vi "AWG Commit.vi"(8 "error in":errorcluster, 11 "Semiconductor Module Context In":T1) -> (0 "error out":errorcluster, 2 "Instruments Handle Out":refnum<k15>[](array[refnum]), 3 "Semiconductor Module Context Out":T1)   [LabVIEW 2013]
uses:
  <vilib>/NI_TestStand_SemiconductorModule/NI_TestStand_Semiconductor_Module.lvlibp/PinMap/General/SemiconductorModuleContext.ctl
  <vilib>/NI_TestStand_SemiconductorModule/NI_TestStand_Semiconductor_Module.lvlibp
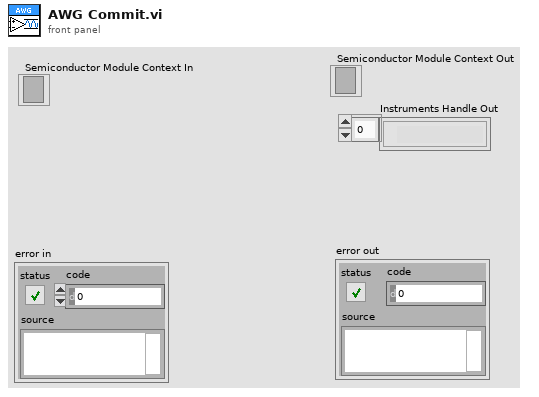
[diagram p1: front panel]
types:
  T1 = typedef "NI_TestStand_Semiconductor_Module.lvlibp/SemiconductorModuleContext.ctl" = refnum<k7>
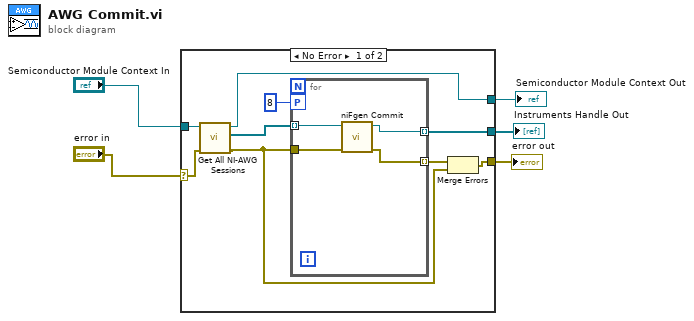
[diagram p0: block diagram]
diagram:
  n1 = case shown="No Error" "error in" {
    selector: "error in" -> [w9 w19]
    tunnel: "Semiconductor Module Context In" -> [w10 _]
    tunnel: [w14 w19] -> w4
    tunnel: [w7 _] -> w3
    tunnel: [w12 _] -> w1
    frame No Error {
      n2 = call "Get All NI-AWG Sessions.vi"("error in (no error)"=w9, "Semiconductor Module Context"=w10) -> ("error out"=w6:errorcluster, "Instrument Sessions"=w8:refnum<k15>[], "Semiconductor Module Context Out"=w7:T1)  [unwired: 7 in]
      n3 = for {
        tunnel: w6 -> [w17]
        tunnel: w8 -> [w18] mode=indexing
        workers-P: 8 -> [_]
        tunnel: [w16] -> w12 mode=indexing
        tunnel: [w15] -> w11 mode=indexing
        n4 = call <instrlib>:"niFgen Commit.vi"("error in (no error)"=w17, "Instrument Handle"=w18) -> ("error out"=w15:errorcluster, "Instrument Handle Out"=w16:refnum<k15>)  [unwired: 8 in]
      }
      n5 = Merge Errors(w11, w6) -> (w14:errorcluster)
    }
    frame Error {
    }
  }
  "error out" <- w4
  "Instruments Handle Out" <- w1
  "Semiconductor Module Context Out" <- w3
